vi "WPI_AnalogChannelGetValue.vi"(8 "error in (no error)":errorcluster, 11 "AIDeviceRef":T1={"DevStatus"={"status"=FALSE, "code"=0, "source"=""}, "Analog Channel"=enum."AI 1"}) -> (0 "error out":errorcluster, 2 "Value":i16, 3 "AIDeviceRef":T1={"DevStatus"={"status"=FALSE, "code"=0, "source"=""}, "Analog Channel"=enum."AI 1"})   [LabVIEW 2017]
doc: "Returns the value of the unscaled analog-to-digital converter (ADC) codes directly from the FPGA. The ADC codes are the binary values that the analog to digital converter returns. The GetVoltage VI references this VI to scale the obtained value into volts.\n\nThis software is licensed. Open the labview\\readme\\WPI Robotics Library Open Source License.txt file for more information."
uses:
  <vilib>/Rock Robotics/WPI/AnalogChannel/WPI_AnalogChannelDevRef.ctl
  <vilib>/Rock Robotics/SystemInterfaces/AI/FPGA_AIChannel.ctl
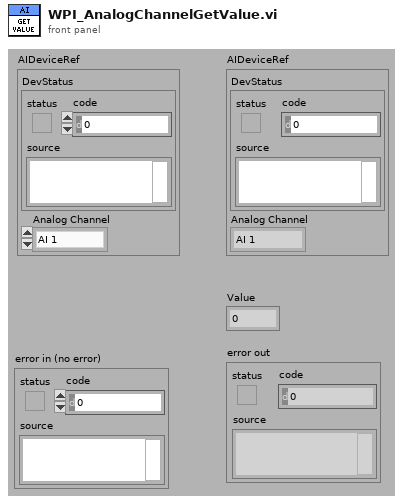
[diagram p1: front panel]
types:
  T1 = typedef "WPI_AnalogChannelDevRef.ctl" = cluster{"DevStatus":errorcluster, "Analog Channel":T2}
  T2 = typedef "FPGA_AIChannel.ctl" = enum8{"AI 0", "AI 1", "AI 2", "AI 3", "AI MXP 0", "AI MXP 1", "AI MXP 2", "AI MXP 3", "Invalid"}
  T3 = typedef "WPI_AnalogModuleDevStatus.ctl" = cluster{"DevStatus":errorcluster}
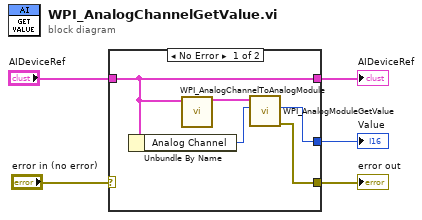
[diagram p0: block diagram]
diagram:
  n1 = case shown="No Error" "error in (no error)" {
    selector: "error in (no error)" -> [_ w12]
    tunnel: "AIDeviceRef" -> [w6 w11]
    tunnel: [w6 w11] -> w4
    tunnel: [w10 _] -> w2
    tunnel: [w7 w12] -> w1
    frame No Error {
      n2 = Unbundle By Name(w6) -> ("Analog Channel"=w8:T2)
      n3 = call <vilib>:"WPI_AnalogChannelToAnalogModule.vi"("AIDeviceRef"=w6) -> ("AIDeviceRef"=w9:T3)  [unwired: 10 out]
      n4 = call <vilib>:"WPI_AnalogModuleGetValue.vi"("Channel"=w8, "AnalogModuleDevRef"=w9) -> ("error out"=w7:errorcluster, "Value"=w10:i32)  [unwired: 1 in, 7 out]
    }
    frame Error {
    }
  }
  "AIDeviceRef" <- w4
  "error out" <- w1
  "Value" <- w2
